vi "ParseInputs.vi"(8 "error in (no error)":errorcluster, 11 "IO.lvclass":refnum<class "IO.lvclass">) -> (0 "error out":errorcluster, 2 "DigitalInput":bool[](array[boolean]), 3 "data":waveform(dbl)[](graph))   [LabVIEW 2018, in "IO.lvclass"]
uses:
  IO.lvclass
  IO.lvclass/IO.ctl
  <vilib>/DAQmx/read.llb/DAQmx Read (Analog 1D Wfm NChan NSamp).vi
  b6b29486-7729-4ab7-b807-ff0c002050a2.vi
  <vilib>/DAQmx/read.llb/DAQmx Read (Digital 1D Bool NChan 1Samp 1Line).vi
  c7f8518d-048a-4bf5-a4a0-0fdd76063358.vi
  <vilib>/DAQmx/miscellaneous.llb/DAQmx Fill In Error Info.vi
  <vilib>/measure/madcrms.llb/Basic Averaged DC-RMS for 1 Chan.vi
  <vilib>/measure/NI_MAPro.lvlib
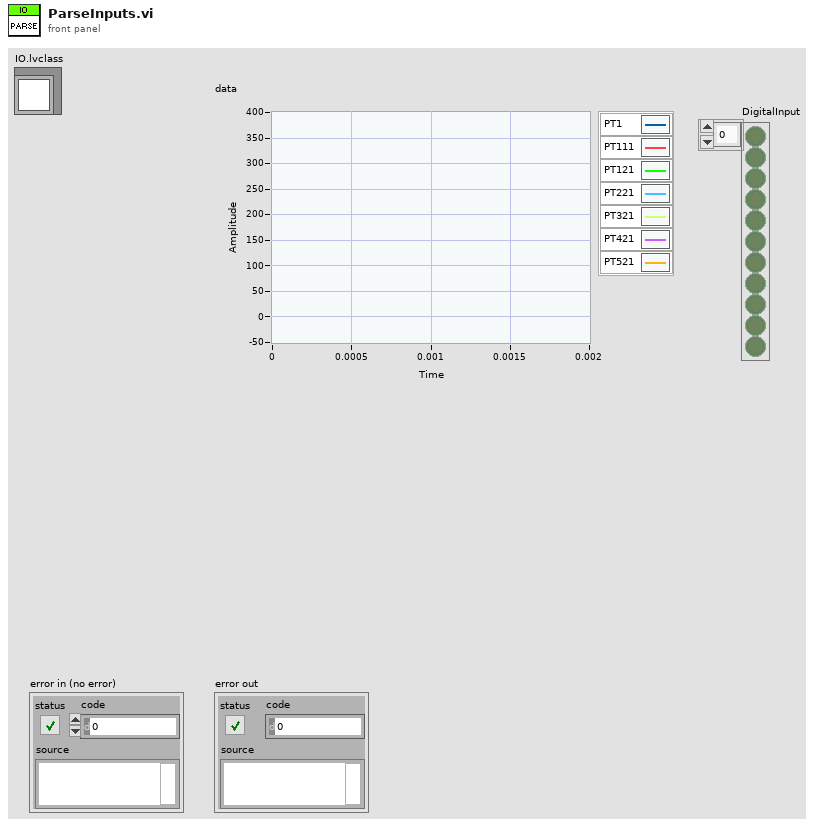
[diagram p1: front panel]
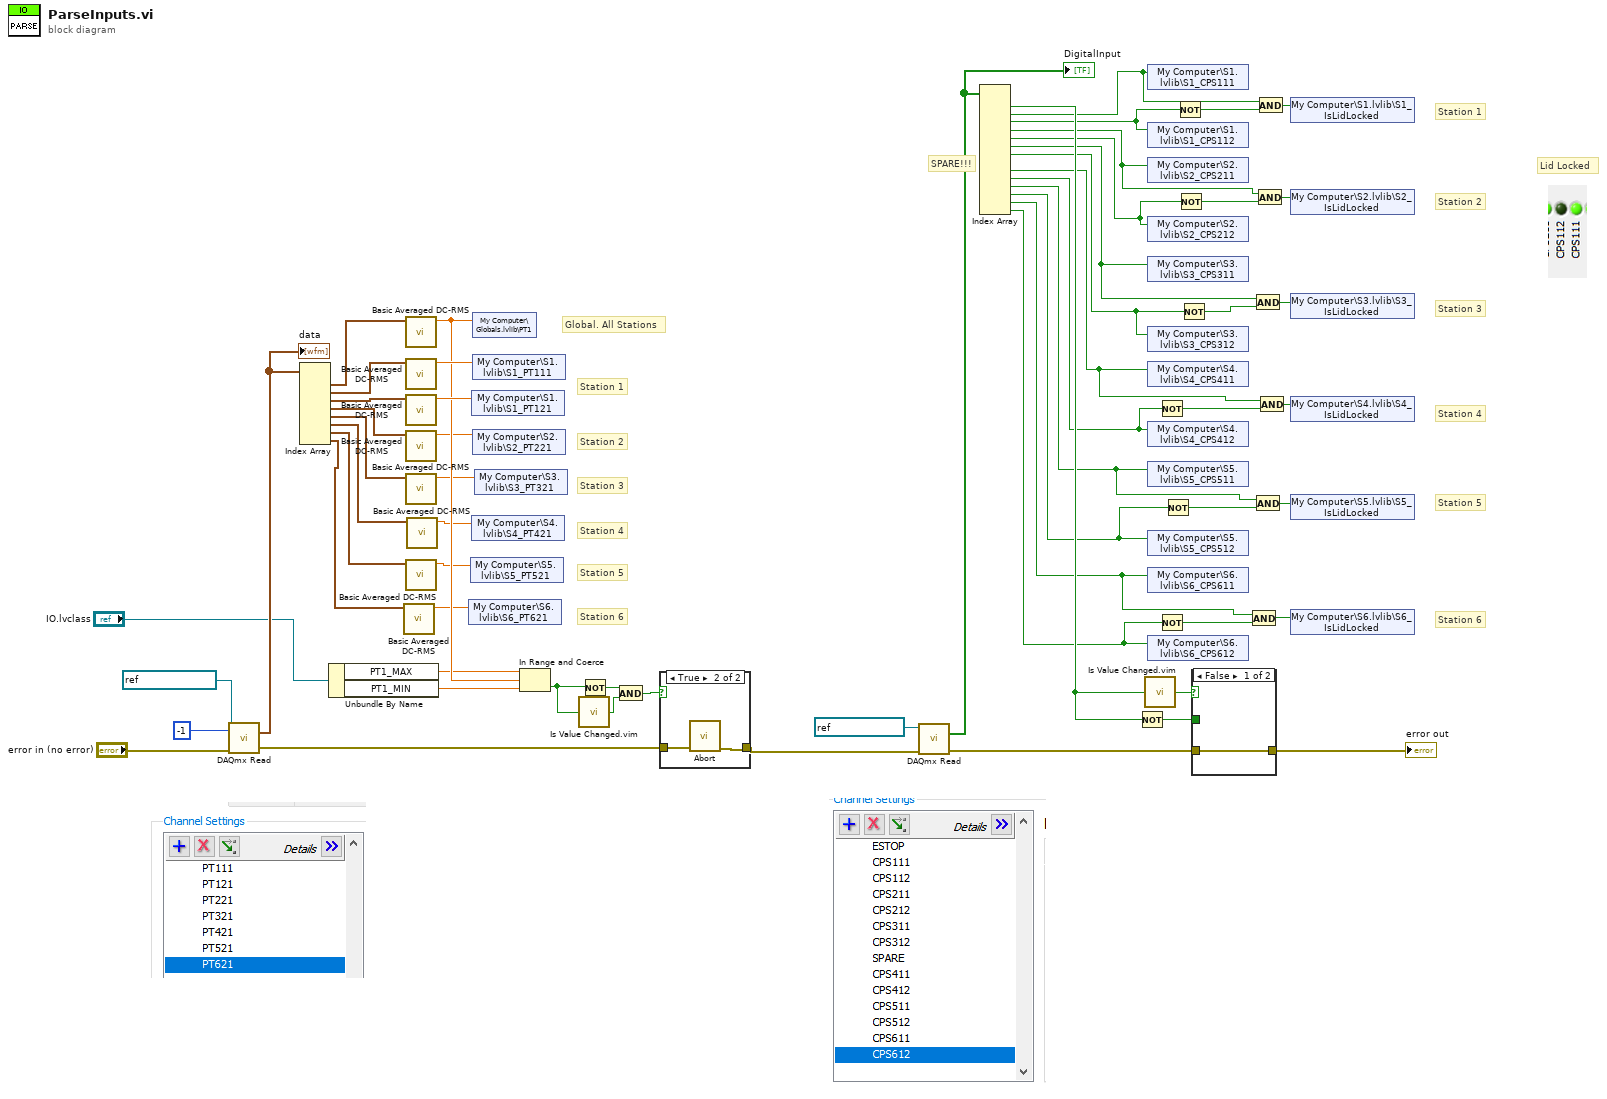
[diagram p0: block diagram]
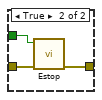
[diagram p3: hidden frame]
diagram:
  # "Station 6"
  # "Station 5"
  # "Station 4"
  # "Station 3"
  # "SPARE!!!"
  # "Station 6"
  # "Station 5"
  # "Station 4"
  # "Station 3"
  # "Lid Locked"
  # "Station 2"
  # "Station 2"
  # "Global. All Stations"
  # "Station 1"
  # "Station 1"
  n1 = call-poly <vilib>:"DAQmx Read.vi"("task/channels in"=refnum<k21> "AnalogInput", "number of samples per channel"=-1, "error in"="error in (no error)") -> ("data"=w59:waveform(dbl)[], "error out"=w36:errorcluster)  [unwired: 10 in, 1 out]
  "data" <- w59
  n2 = Index Array(array=w59) -> (element #1=w42:waveform(dbl), element #2=w43:waveform(dbl), element #3=w44:waveform(dbl), element #4=w34:waveform(dbl), element #5=w24:waveform(dbl), element #6=w22:waveform(dbl), element #7=w18:waveform(dbl), element #8=w17:waveform(dbl))  [unwired: 8 in]
  n3 = Unbundle By Name("IO.lvclass") -> ("PT1_MAX"=w26:dbl, "PT1_MIN"=w25:dbl)
  n4 = call-poly <vilib>:"Basic Averaged DC-RMS.vi"("signal in"=w17) -> ("DC value"=w19:dbl)  [unwired: 7 in, 3 out]
  n5 = call-poly <vilib>:"Basic Averaged DC-RMS.vi"("signal in"=w42) -> ("DC value"=w41:dbl)  [unwired: 7 in, 3 out]
  n6 = call-poly <vilib>:"Basic Averaged DC-RMS.vi"("signal in"=w43) -> ("DC value"=w60:dbl)  [unwired: 7 in, 3 out]
  n7 = call-poly <vilib>:"Basic Averaged DC-RMS.vi"("signal in"=w44) -> ("DC value"=w54:dbl)  [unwired: 7 in, 3 out]
  n8 = call-poly <vilib>:"Basic Averaged DC-RMS.vi"("signal in"=w34) -> ("DC value"=w33:dbl)  [unwired: 7 in, 3 out]
  n9 = call-poly <vilib>:"Basic Averaged DC-RMS.vi"("signal in"=w24) -> ("DC value"=w23:dbl)  [unwired: 7 in, 3 out]
  n10 = call-poly <vilib>:"Basic Averaged DC-RMS.vi"("signal in"=w18) -> ("DC value"=w20:dbl)  [unwired: 7 in, 3 out]
  n11 = call-poly <vilib>:"Basic Averaged DC-RMS.vi"("signal in"=w22) -> ("DC value"=w21:dbl)  [unwired: 7 in, 3 out]
  n12 = shared-variable "My Computer\\S6.lvlib\\S6_PT621"(w19) -> ()  [unwired: 1 in, 1 out]
  n13 = shared-variable "My Computer\\S5.lvlib\\S5_PT521"(w20) -> ()  [unwired: 1 in, 1 out]
  n14 = shared-variable "My Computer\\S1.lvlib\\S1_PT121"(w54) -> ()  [unwired: 1 in, 1 out]
  n15 = shared-variable "My Computer\\S4.lvlib\\S4_PT421"(w21) -> ()  [unwired: 1 in, 1 out]
  n16 = shared-variable "My Computer\\Globals.lvlib\\PT1"(w41) -> ()  [unwired: 1 in, 1 out]
  n17 = shared-variable "My Computer\\S1.lvlib\\S1_PT111"(w60) -> ()  [unwired: 1 in, 1 out]
  n18 = shared-variable "My Computer\\S2.lvlib\\S2_PT221"(w33) -> ()  [unwired: 1 in, 1 out]
  n19 = shared-variable "My Computer\\S3.lvlib\\S3_PT321"(w23) -> ()  [unwired: 1 in, 1 out]
  n20 = In Range and Coerce(upper limit=w26, x=w41, lower limit=w25) -> (In Range?=w39:bool)  [unwired: 1 out]
  n21 = call "Is Value Changed.vim"("value"=w39) -> ("changed or first call?"=w40:bool)
  n22 = Not(x=w39) -> (.not. x?=w38:bool)
  n23 = And(x=w38, y=w40) -> (x .and. y?=w37:bool)
  n24 = case shown="True" w37 {
    tunnel: w36 -> [w61 w63]
    tunnel: [w61 w62] -> w35
    frame False {
    }
    frame True {
      n25 = call "Abort.vi"("error in"=w63) -> ("error out"=w62:errorcluster)  [unwired: 10 in]
    }
  }
  n26 = call-poly <vilib>:"DAQmx Read.vi"("task/channels in"=refnum<k21> "DigitalInput", "error in"=w35) -> ("data"=w53:bool[], "error out"=w52:errorcluster)  [unwired: 11 in, 1 out]
  "DigitalInput" <- w53
  n27 = Index Array(array=w53) -> (element #1=w50:bool, element #2=w47:bool, element #3=w46:bool, element #4=w32:bool, element #5=w31:bool, element #6=w14:bool, element #7=w15:bool, element #9=w9:bool, element #10=w10:bool, element #11=w7:bool, element #12=w8:bool, element #13=w2:bool, element #14=w3:bool)  [unwired: 14 in, 1 out]
  n28 = Not(x=w50) -> (.not. x?=w48:bool)
  n29 = call "Is Value Changed.vim"("value"=w50) -> ("changed or first call?"=w49:bool)
  n30 = shared-variable "My Computer\\S1.lvlib\\S1_CPS111"(w47) -> ()  [unwired: 1 in, 1 out]
  n31 = shared-variable "My Computer\\S1.lvlib\\S1_CPS112"(w46) -> ()  [unwired: 1 in, 1 out]
  n32 = shared-variable "My Computer\\S2.lvlib\\S2_CPS211"(w32) -> ()  [unwired: 1 in, 1 out]
  n33 = shared-variable "My Computer\\S2.lvlib\\S2_CPS212"(w31) -> ()  [unwired: 1 in, 1 out]
  n34 = shared-variable "My Computer\\S3.lvlib\\S3_CPS311"(w14) -> ()  [unwired: 1 in, 1 out]
  n35 = shared-variable "My Computer\\S3.lvlib\\S3_CPS312"(w15) -> ()  [unwired: 1 in, 1 out]
  n36 = shared-variable "My Computer\\S4.lvlib\\S4_CPS411"(w9) -> ()  [unwired: 1 in, 1 out]
  n37 = shared-variable "My Computer\\S4.lvlib\\S4_CPS412"(w10) -> ()  [unwired: 1 in, 1 out]
  n38 = shared-variable "My Computer\\S5.lvlib\\S5_CPS511"(w7) -> ()  [unwired: 1 in, 1 out]
  n39 = shared-variable "My Computer\\S5.lvlib\\S5_CPS512"(w8) -> ()  [unwired: 1 in, 1 out]
  n40 = shared-variable "My Computer\\S6.lvlib\\S6_CPS611"(w2) -> ()  [unwired: 1 in, 1 out]
  n41 = shared-variable "My Computer\\S6.lvlib\\S6_CPS612"(w3) -> ()  [unwired: 1 in, 1 out]
  n42 = Not(x=w10) -> (.not. x?=w11:bool)
  n43 = Not(x=w3) -> (.not. x?=w4:bool)
  n44 = Not(x=w8) -> (.not. x?=w6:bool)
  n45 = Not(x=w46) -> (.not. x?=w29:bool)
  n46 = Not(x=w31) -> (.not. x?=w28:bool)
  n47 = Not(x=w15) -> (.not. x?=w16:bool)
  n48 = case shown="False" w49 {
    tunnel: w52 -> [w64 w67]
    tunnel: [w64 w66] -> w51
    tunnel: w48 -> [_ w65]
    frame False {
    }
    frame True {
      n49 = call "Estop.vi"("error in"=w67, "ESTOP"=w65) -> ("error out"=w66:errorcluster)  [unwired: 9 in]
    }
  }
  "error out" <- w51
  n50 = And(x=w2, y=w4) -> (x .and. y?=w1:bool)
  n51 = And(x=w14, y=w16) -> (x .and. y?=w13:bool)
  n52 = And(x=w7, y=w6) -> (x .and. y?=w5:bool)
  n53 = And(x=w32, y=w28) -> (x .and. y?=w30:bool)
  n54 = And(x=w47, y=w29) -> (x .and. y?=w45:bool)
  n55 = And(x=w9, y=w11) -> (x .and. y?=w12:bool)
  n56 = shared-variable "My Computer\\S1.lvlib\\S1_IsLidLocked"(w45) -> ()  [unwired: 1 in, 1 out]
  n57 = shared-variable "My Computer\\S2.lvlib\\S2_IsLidLocked"(w30) -> ()  [unwired: 1 in, 1 out]
  n58 = shared-variable "My Computer\\S3.lvlib\\S3_IsLidLocked"(w13) -> ()  [unwired: 1 in, 1 out]
  n59 = shared-variable "My Computer\\S4.lvlib\\S4_IsLidLocked"(w12) -> ()  [unwired: 1 in, 1 out]
  n60 = shared-variable "My Computer\\S5.lvlib\\S5_IsLidLocked"(w5) -> ()  [unwired: 1 in, 1 out]
  n61 = shared-variable "My Computer\\S6.lvlib\\S6_IsLidLocked"(w1) -> ()  [unwired: 1 in, 1 out]
